vi "LbcbConversions.vi"(7 "LbcbConversionType":T3, 8 "error in (no error)":errorcluster, 9 "Inputs":dbl[](array[numeric]), 10 "LBCB Number":T2, 11 "ConversionOps":T1(ring)) -> (0 "error out":errorcluster, 1 "Outputs":dbl[](array[numeric]))   [LabVIEW 2013]
uses:
  LbcbConversionTypes.ctl
  Data Access Objects/Metadata/LBCB Number.ctl
  Data Access Objects/Metadata/DAO Actions with Remove.ctl
  C:/Users/mbletzin/Desktop/Work/NewLbcbConversionDll/DLL/LbcbConversions.dll
  DLL/LbcbConversions.dll
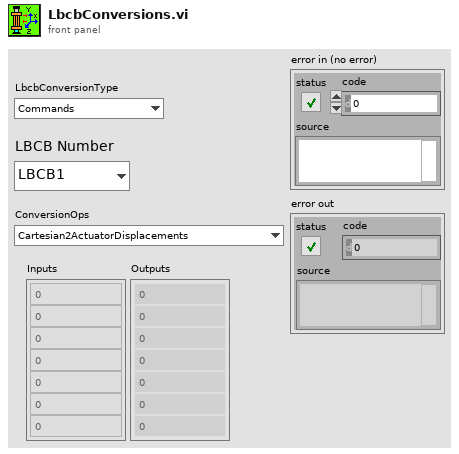
[diagram p1: front panel]
types:
  T1 = enum16{"Cartesian2ActuatorDisplacements", "Actuator2CartesianDisplacements", "Actuators2CartesianForces"}
  T2 = typedef "LBCB Number.ctl" = enum16{"LBCB1", "LBCB2"}
  T3 = typedef "LbcbConversionTypes.ctl" = enum16{"Commands", "Readings", "Offsets"}
  T4 = typedef "DAO Actions with Remove.ctl" = enum16{"Init", "Get", "Set", "Remove"}
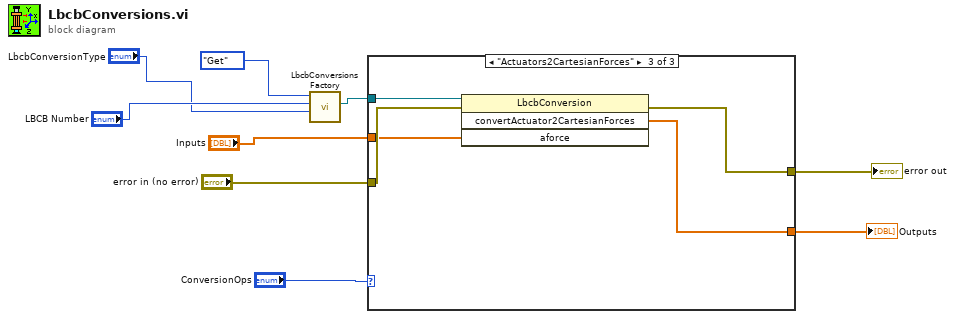
[diagram p0: block diagram]
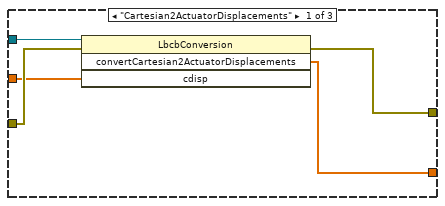
[diagram p2: hidden frame]
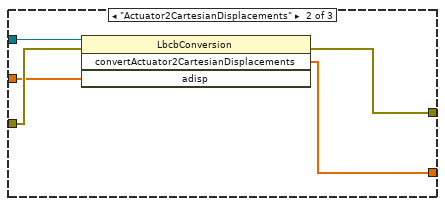
[diagram p3: hidden frame]
diagram:
  n1 = call "LbcbConversionsFactory.vi"("LbcbConversionType"="LbcbConversionType", "LBCB Number"="LBCB Number", "Actions"=DAO_Actions_with_Remove."Get") -> ("Conversion Ref"=w5:refnum<k24>)  [unwired: 7 in, 1 out]
  n2 = case shown="\"Actuators2CartesianForces\"" "ConversionOps" {
    tunnel: w5 -> [w14 w19 w24]
    tunnel: "error in (no error)" -> [w13 w18 w23]
    tunnel: [w12 w17 w22] -> w3
    tunnel: "Inputs" -> [w11 w16 w21]
    tunnel: [w10 w15 w20] -> w1
    frame "Cartesian2ActuatorDisplacements" {
      n3 = invoke class="LbcbConversion" method="convertCartesian2ActuatorDisplacements"(reference=w14, error in=w13, "cdisp"=w11) -> (error out=w12:errorcluster, "convertCartesian2ActuatorDisplacements"=w10:dbl[])  [unwired: 1 in, 2 out]
    }
    frame "Actuator2CartesianDisplacements" {
      n4 = invoke class="LbcbConversion" method="convertActuator2CartesianDisplacements"(reference=w19, error in=w18, "adisp"=w16) -> (error out=w17:errorcluster, "convertActuator2CartesianDisplacements"=w15:dbl[])  [unwired: 1 in, 2 out]
    }
    frame "Actuators2CartesianForces" {
      n5 = invoke class="LbcbConversion" method="convertActuator2CartesianForces"(reference=w24, error in=w23, "aforce"=w21) -> (error out=w22:errorcluster, "convertActuator2CartesianForces"=w20:dbl[])  [unwired: 1 in, 2 out]
    }
  }
  "Outputs" <- w1
  "error out" <- w3
